vi "Activity Log.vi"(6 "Log File Path":path, 7 "Action":T1, 8 "Error In":errorcluster, 9 "string ref":refnum<vi>, 11 "Message Log Entry":string) -> (0 "Error Out":errorcluster, 2 "rows":i32, 3 "Message Log":string)   [LabVIEW 2024]
doc: "This functional global timestamps and records text messages for a generic message log."
uses:
  Activity Log enum Action .ctl
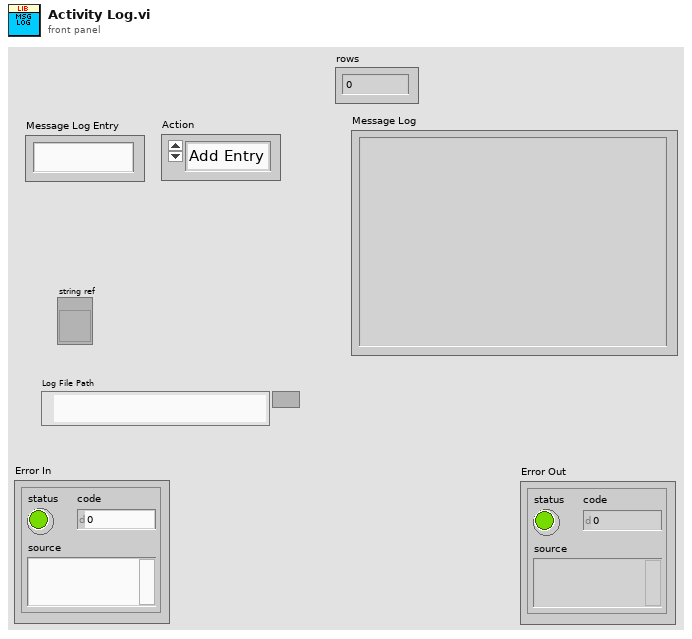
[diagram p1: front panel]
types:
  T1 = typedef "Activity Log enum Action .ctl" = enum16{"Add Entry", "Get Log", "Restore From Disk", "Save to Disk", "Init", "Clear"}
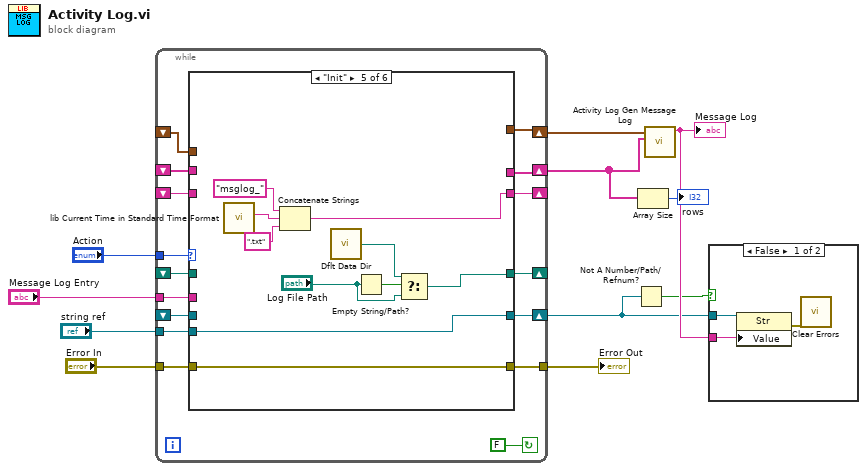
[diagram p0: block diagram]
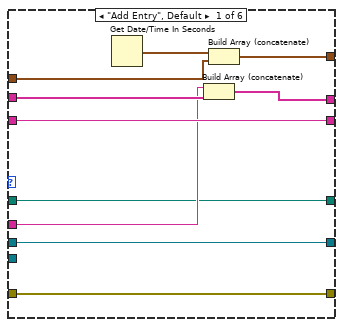
[diagram p3: hidden frame]
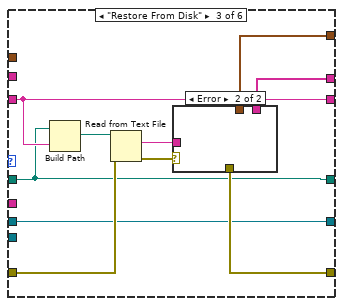
[diagram p5: hidden frame]
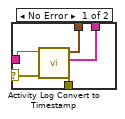
[diagram p6: hidden frame]
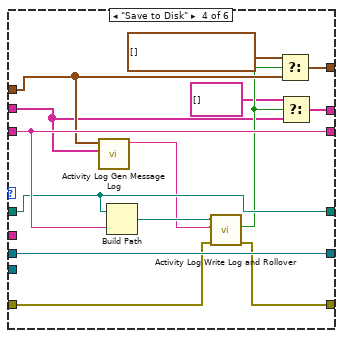
[diagram p7: hidden frame]
diagram:
  n1 = while {
    tunnel: "Action" -> [w27]
    shift-right: [w23] -> w7
    shift-left: _ -> [w22]
    shift-right: [w24] -> w2
    shift-left: _ -> [w21]
    tunnel: "Message Log Entry" -> [w25]
    tunnel: "Error In" -> [w20]
    tunnel: [w19] -> w8
    shift-right: [w18] -> _
    shift-left: _ -> [w17]
    shift-right: [w16] -> w4
    shift-left: _ -> [w14]
    tunnel: "string ref" -> [w15]
    shift-right: [w13] -> _
    shift-left: _ -> [w12]
    stop <- FALSE continue-if-true
    n2 = case shown="\"Init\"" w27 {
      tunnel: w25 -> [w31 _ _ _ _ _]
      tunnel: [w37 w43 w48 w60 _ _] -> w24
      tunnel: [w36 w42 w49 w63 _ _] -> w23
      tunnel: w22 -> [w30 w42 _ w65 _ _]
      tunnel: w21 -> [w35 w43 _ w61 _ _]
      tunnel: w20 -> [w34 w41 w51 w69 w82 w86]
      tunnel: [w34 w41 w50 w68 w82 w86] -> w19
      tunnel: [w33 w40 w47 w72 w73 w83] -> w18
      tunnel: w17 -> [w33 w40 w47 w72 _ w83]
      tunnel: [w32 w39 w46 w71 w81 w85] -> w16
      tunnel: w15 -> [_ _ _ _ w81 _]
      tunnel: w14 -> [w32 w39 w46 w71 _ w85]
      tunnel: [w28 w38 w45 w70 w77 w84] -> w13
      tunnel: w12 -> [w28 w38 w45 w70 _ w84]
      frame "Add Entry", Default {
        n3 = Get Date/Time In Seconds() -> (seconds since 1Jan1904=w29:timestamp)
        n4 = Build Array (concatenate)(w31, w35) -> (w37:string[])
        n5 = Build Array (concatenate)(w29, w30) -> (w36:timestamp[])
      }
      frame "Get Log" {
      }
      frame "Restore From Disk" {
        n6 = Build Path(base path=w45, name or relative path=w47) -> (appended path=w53:path)
        n7 = Read from Text File(file (use dialog)=w53, error in=w51) -> (text=w52:string, error out=w44:errorcluster)  [unwired: 2 in, 2 out]
        n8 = case shown="Error" w44 {
          selector: w44 -> [w54 _]
          tunnel: w52 -> [w58 _]
          tunnel: [w57 _] -> w50
          tunnel: [w56 _] -> w49
          tunnel: [w55 _] -> w48
          frame No Error {
            n9 = call "Activity Log Convert to Timestamp.vi"("error in (no error)"=w54, "Message Log"=w58) -> ("error out"=w57:errorcluster, "Messages"=w55:string[], "timestamps"=w56:timestamp[])  [unwired: 7 in]
          }
          frame Error {
          }
        }
      }
      frame "Save to Disk" {
        n10 = call "Activity Log Gen Message Log.vi"("Messages"=w61, "Timestamps"=w65) -> ("Message Log"=w66:string)  [unwired: 8 in, 1 out]
        n11 = Build Path(base path=w70, name or relative path=w72) -> (appended path=w67:path)
        n12 = call "Activity Log Write Log and Rollover.vi"("error in (no error)"=w69, "Log Text"=w66, "Log File"=w67) -> ("error out"=w68:errorcluster, "new file?"=w62:bool)  [unwired: 6 in, 1 out]
        n13 = Select(t=timestamp[] [], s=w62, f=w65) -> (s? t:f=w63:timestamp[])
        n14 = Select(t=string[] [], s=w62, f=w61) -> (s? t:f=w60:string[])
      }
      frame "Init" {
        n15 = call "lib Current Time in Standard Time Format.vi"() -> ("date/time string"=w76:string)  [unwired: 11 in]
        n16 = Concatenate Strings("msglog_" ("string"), w76, ".txt" ("string")) -> (w73:string)
        n17 = call <vilib>:"Dflt Data Dir.vi"() -> ("App:Default Data Directory"=w78:path)
        n18 = Empty String/Path?(string/path="Log File Path") -> (empty?=w80:bool)
        n19 = Select(t=w78, s=w80, f="Log File Path") -> (s? t:f=w77:path)
      }
      frame "Clear" {
      }
    }
  }
  "Error Out" <- w8
  n20 = Not A Number/Path/Refnum?(number/path/refnum=w4) -> (NaN/Path/Refnum?=w3:bool)
  n21 = Array Size(array=w2) -> (size(s)=→"rows":i32)
  n22 = call "Activity Log Gen Message Log.vi"("Messages"=w2, "Timestamps"=w7) -> ("Message Log"=w5:string)  [unwired: 8 in, 1 out]
  "Message Log" <- w5
  n23 = case shown="False" w3 {
    tunnel: w5 -> [w89 _]
    tunnel: w4 -> [w88 _]
    frame False {
      n24 = property class="Str"(reference=w88, "Value"=w89) -> (error out=w87:errorcluster)  [unwired: 1 in, 1 out]
      n25 = call <vilib>:"Clear Errors.vi"("error in (no error)"=w87) -> ()  [unwired: 5 in, 2 out]
    }
    frame True {
    }
  }
